vi "RouteGuide RouteChat.vi"(3 "error in (no error)":errorcluster, 4 "gRPCid in":T1, 5 "DNL_LabVIEW Object in":refnum<class "RouteGuideImpl.lvclass">) -> (0 "error out":errorcluster, 1 "gRPCid out":T1, 2 "DNL_LabVIEW Object out":refnum<class "RouteGuideImpl.lvclass">)   [LabVIEW 2019, in "UserCode_server.lvlib" / "RouteGuideImpl.lvclass"]
uses:
  RouteGuideImpl.lvclass
  <vilib>/gRPC/LabVIEW gRPC Library/Shared/grpcId.ctl
  Generated_server/RPC Service/RouteGuide/RouteGuide.lvclass
  <vilib>/gRPC/LabVIEW gRPC Library/grpc-lvsupport-release.lvlib
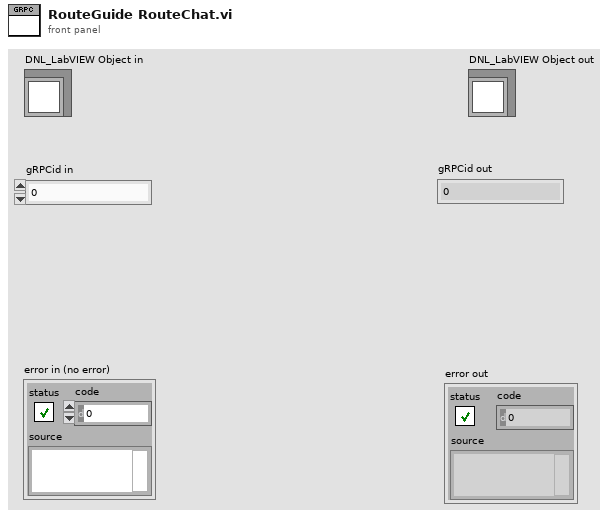
[diagram p1: front panel]
types:
  T1 = typedef "grpc-lvsupport-release.lvlib/grpcId.ctl" = u64
  T2 = typedef "Generated_server.lvlib/routeguide_RouteNote.ctl" = cluster{"location":T3, "message":string}
  T3 = typedef "Generated_server.lvlib/routeguide_Point.ctl" = cluster{"latitude":i32, "longitude":i32}
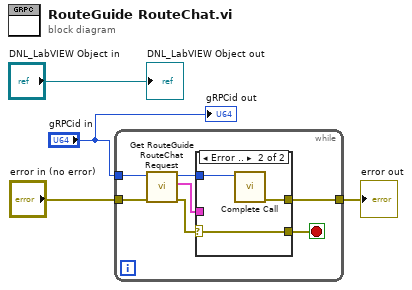
[diagram p0: block diagram]
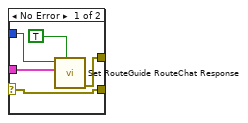
[diagram p2: hidden frame]
diagram:
  n1 = while {
    tunnel: "gRPCid in" -> [w7]
    tunnel: "error in (no error)" -> [w6]
    tunnel: [w5] -> w3
    stop <- w11 stop-if-true
    n2 = call "Get RouteGuide RouteChat Request.vi"("error in (no error)"=w6, "gRPCid"=w7) -> ("error out"=w8:errorcluster, "Message Data"=w9:T2, "gRPCid out"=w10:T1)  [unwired: 7 in]
    n3 = case shown="Error .." w8 {
      selector: w8 -> [w16 w19]
      tunnel: w10 -> [w15 w18]
      tunnel: w9 -> [w14 _]
      tunnel: [w16 w19] -> w11
      tunnel: [w12 w17] -> w5
      frame No Error {
        n4 = call "Set RouteGuide RouteChat Response.vi"("Streaming? (F)"=TRUE ("Streeming? (F)"), "Message Data"=w14, "gRPCid in"=w15) -> ("error out"=w12:errorcluster)  [unwired: 8 in]
      }
      frame Error {
        n5 = call <vilib>:"Complete Call.vi"("gRPCid"=w18) -> ("error out"=w17:errorcluster)  [unwired: 9 in]
      }
    }
  }
  "error out" <- w3
  "DNL_LabVIEW Object out" <- "DNL_LabVIEW Object in"
  "gRPCid out" <- "gRPCid in"
